vi "2D_tipconvolution.vi"() -> ()   [LabVIEW 2017]
uses:
  <vilib>/Analysis/2dsp.llb/2D Real FFT.vi
  <vilib>/Analysis/2dsp.llb/2D Inverse Real FFT.vi
  <vilib>/Analysis/NI_AALBase.lvlib
  <vilib>/Analysis/NI_AALPro.lvlib
panel:
  out "II tip sample convolution":dbl[][](graph)
  in  "index (row)":i32=18
  out "Sample crossections":dynamicdata(graph)
  out "tip sample convolution":dbl[][](graph)
  in  "tipangle":dbl=20.0 min=1.0 max=89.0 format="%.2f"
  in  "radius of curvature":dbl=10.0 min=-0.0 max=1000.0 format="%.2f"
  out "tipshape crossection horizontal":dbl[](graph)=[0.0, 0.0, 0.0, 0.0, 0.0, 0.0, 0.0, 0.0, 0.0, 0.0, 0.0, 0.0, 0.0, 0.0, 0.0, 0.0, 0.0, 0.0, 0.0, 0.0, 0.0, 0.0, 0.0, 0.0, 0.0, 0.0, 0.0, 0.0, 0.0, 0.0, 0.0, 0.0, 0.0, 0.0, 0.0, 0.0, 0.0, 0.0, 0.0, 0.0, 0.0, 0.0, 0.0, 0.0, 0.0, 0.0, 0.0, 0.0, 0.0, 0.0, 0.0, 0.0, 0.0, 0.0, 0.0, 0.0, 0.0, 0.0, 0.0, 0.0, 0.0, 0.0, 0.0, 0.0, 0.0, 0.0, 0.0, 0.0, 0.0, 0.0, 0.0, 0.0, 0.0, 0.0, 0.0, 0.0, 0.0, 0.0, 0.0, 0.0, 0.0, 0.0, 0.0, 0.0, 0.0, 0.0, 0.0, 0.0, 0.0, 0.0, 0.0, 0.0, 0.0, 0.0, 0.0, 0.0, 0.0, 0.0, 0.0, 0.0, 0.0, 0.0, 0.0, 0.0, 0.0, 0.0, 0.0, 0.0, 0.0, 0.0, 0.0, 0.0, 0.0, 0.0, 0.0, 0.0, 0.0, 0.0, 0.0, 0.0, 0.0, 0.0, 0.0, 0.0, 0.0, 0.0, 0.0, 0.0, 0.0, 0.0, 0.0, 0.0, 0.0, 0.0, 0.0, 0.0, 0.0, 0.0, 0.0, 0.0, 0.0, 0.0, 0.0, 0.0, 0.0, 0.0, 0.0, 0.0, 0.0, 0.0, 0.0, 0.0, 0.0, 0.0, 0.0, 0.0, 0.0, 0.0, 0.0, 0.0, 0.0, 0.0, 0.0, 0.0, 0.0, 0.0, 0.0, 0.0, 0.0, 0.0, 0.0, 0.0, 0.0, 0.0, 0.0, 0.0, 0.0, 0.0, 0.0, 0.0, 0.0, 0.0, 0.0, 0.0, 0.0, 0.0, 0.0, 0.0, 0.0, 0.0, 0.0, 0.0, 0.0, 0.0, 0.0, 0.0, 0.0, 0.0, 0.0, 0.0, 0.0, 0.0, 0.0, 0.0, 0.0, 0.0, 0.0, 0.0, 0.0, 0.0, 0.0, 0.0, 0.0, 0.0, 0.0, 0.0, 0.0, 0.0, 0.0, 0.0, 0.0, 0.0, 0.0, 0.0, 0.0, 0.0, 0.0, 0.0, 0.0, 0.0, 0.0, 0.0, 0.0, 0.0, 0.0, 0.0, 0.0, 0.0, 0.0, 1.7632698070846526, 4.358898943540674, 6.0, 7.14142842854285, 8.0, 8.660254037844387, 9.16515138991168, 9.539392014169456, 9.797958971132712, 9.9498743710662, 10.0, 9.9498743710662, 10.0, 9.9498743710662, 9.797958971132712, 9.539392014169456, 9.16515138991168, 8.660254037844387, 8.0, 7.14142842854285, 6.0, 4.358898943540674, 1.7632698070846526, 0.0, 0.0, 0.0, 0.0, 0.0, 0.0, 0.0, 0.0, 0.0, 0.0, 0.0, 0.0, 0.0, 0.0, 0.0, 0.0, 0.0, 0.0, 0.0, 0.0, 0.0, 0.0, 0.0, 0.0, 0.0, 0.0, 0.0, 0.0, 0.0, 0.0, 0.0, 0.0, 0.0, 0.0, 0.0, 0.0, 0.0, 0.0, 0.0, 0.0, 0.0, 0.0, 0.0, 0.0, 0.0, 0.0, 0.0, 0.0, 0.0, 0.0, 0.0, 0.0, 0.0, 0.0, 0.0, 0.0, 0.0, 0.0, 0.0, 0.0, 0.0, 0.0, 0.0, 0.0, 0.0, 0.0, 0.0, 0.0, 0.0, 0.0, 0.0, 0.0, 0.0, 0.0, 0.0, 0.0, 0.0, 0.0, 0.0, 0.0, 0.0, 0.0, 0.0, 0.0, 0.0, 0.0, 0.0, 0.0, 0.0, 0.0, 0.0, 0.0, 0.0, 0.0, 0.0, 0.0, 0.0, 0.0, 0.0, 0.0, 0.0, 0.0, 0.0, 0.0, 0.0, 0.0, 0.0, 0.0, 0.0, 0.0, 0.0, 0.0, 0.0, 0.0, 0.0, 0.0, 0.0, 0.0, 0.0, 0.0, 0.0, 0.0, 0.0, 0.0, 0.0, 0.0, 0.0, 0.0, 0.0, 0.0, 0.0, 0.0, 0.0, 0.0, 0.0, 0.0, 0.0, 0.0, 0.0, 0.0, 0.0, 0.0, 0.0, 0.0, 0.0, 0.0, 0.0, 0.0, 0.0, 0.0, 0.0, 0.0, 0.0, 0.0, 0.0, 0.0, 0.0, 0.0, 0.0, 0.0, 0.0, 0.0, 0.0, 0.0, 0.0, 0.0, 0.0, 0.0, 0.0, 0.0, 0.0, 0.0, 0.0, 0.0, 0.0, 0.0, 0.0, 0.0, 0.0, 0.0, 0.0, 0.0, 0.0, 0.0, 0.0, 0.0, 0.0, 0.0, 0.0, 0.0, 0.0, 0.0, 0.0, 0.0, 0.0, 0.0, 0.0, 0.0, 0.0, 0.0, 0.0, 0.0, 0.0, 0.0, 0.0, 0.0, 0.0, 0.0, 0.0, 0.0, 0.0, 0.0, 0.0, 0.0, 0.0, 0.0, 0.0, 0.0, 0.0, 0.0, 0.0, 0.0, 0.0, 0.0, 0.0, 0.0, 0.0, 0.0, 0.0, 0.0, 0.0, 0.0, 0.0, 0.0, 0.0, 0.0, 0.0, 0.0]
  out "block pattern like the NT-MDT TGQ01":dbl[][](graph)
  in  "cycles y":dbl=5.0 format="%0.2f"
  in  "pixels y":i32=500
  in  "cycles x":dbl=3.0 format="%0.2f"
  in  "pixels x":i32=500
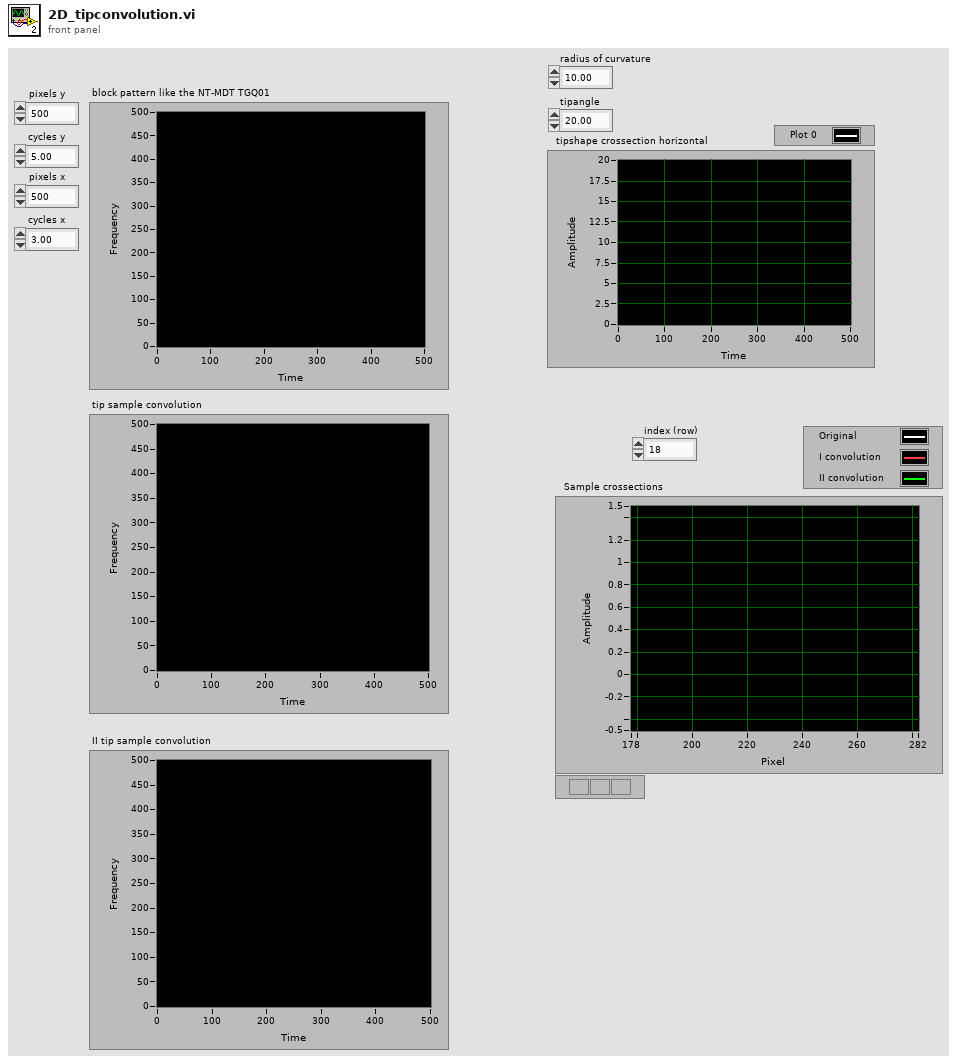
[diagram p1: front panel]
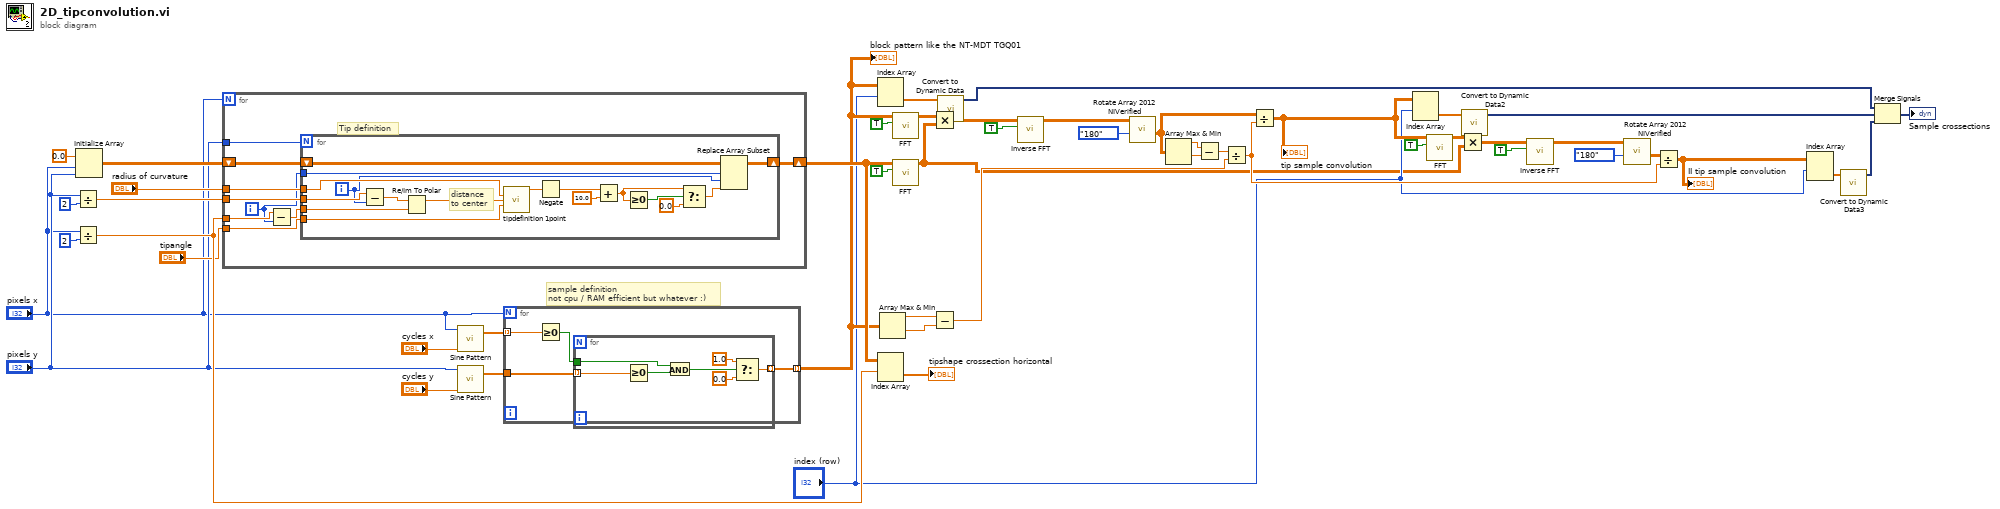
[diagram p0: block diagram]
diagram:
  # "sample definition\nnot cpu / RAM efficient but whatever :)"
  n1 = Divide(x="pixels y", y=2) -> (x/y=w44:dbl)
  n2 = Divide(x="pixels x", y=2) -> (x/y=w43:dbl)
  n3 = Initialize Array(0.0 ("element"), "pixels x", "pixels y") -> (w39:dbl[][])
  n4 = for {
    N: "pixels x" -> [_]
    tunnel: "pixels y" -> [w59]
    tunnel: w43 -> [w57]
    tunnel: w44 -> [w58]
    tunnel: "radius of curvature" -> [w56]
    tunnel: "tipangle" -> [w55]
    shift-right: [w53] -> w33
    shift-left: w39 -> [w54]
    i -> [w52]
    # "Tip definition"
    n5 = Subtract(x=w57, y=w52) -> (x-y=w51:dbl)
    n6 = for {
      N: w59 -> [_]
      tunnel: w58 -> [w76]
      tunnel: w56 -> [w75]
      tunnel: w55 -> [w74]
      shift-right: [w73] -> w53
      shift-left: w54 -> [w72]
      tunnel: w52 -> [w70]
      tunnel: w51 -> [w68]
      i -> [w71]
      # "distance\nto center"
      n7 = Subtract(x=w76, y=w71) -> (x-y=w69:dbl)
      n8 = Re/Im To Polar(2:w68, 3:w69) -> (1:w67:dbl)  [unwired: 1 out]
      n9 = call "tipdefinition 1point.vi"("radius of curvature"=w75, "x"=w67, "tipangle"=w74) -> ("result"=w66:dbl)  [unwired: 12 in]
      n10 = Negate(x=w66) -> (-x=w65:dbl)
      n11 = Add(x=w65, y=10.0) -> (x+y=w62:dbl)
      n12 = Greater Or Equal To 0?(x=w62) -> (x >= 0?=w63:bool)
      n13 = Select(t=w62, s=w63, f=0.0) -> (s? t:f=w60:dbl)
      n14 = Replace Array Subset(array=w72, new element=w60, index (row)=w70, index (col)=w71) -> (w73:dbl[][])
    }
  }
  n15 = call <vilib>:"Sine Pattern.vi"("cycles"="cycles x", "samples"="pixels x") -> ("Sinusoidal Pattern"=w47:dbl[])  [unwired: 2 in, 1 out]
  n16 = call <vilib>:"Sine Pattern.vi"("cycles"="cycles y", "samples"="pixels y") -> ("Sinusoidal Pattern"=w48:dbl[])  [unwired: 2 in, 1 out]
  n17 = for {
    N: "pixels x" -> [_]
    tunnel: w48 -> [w77]
    tunnel: w47 -> [w79] mode=indexing
    tunnel: [w80] -> w16 mode=indexing
    n18 = Greater Or Equal To 0?(x=w79) -> (x >= 0?=w78:bool)
    n19 = for {
      tunnel: w77 -> [w87] mode=indexing
      tunnel: [w84] -> w80 mode=indexing
      tunnel: w78 -> [w83]
      n20 = Greater Or Equal To 0?(x=w87) -> (x >= 0?=w82:bool)
      n21 = And(x=w83, y=w82) -> (x .and. y?=w81:bool)
      n22 = Select(t=1.0, s=w81, f=0.0) -> (s? t:f=w84:dbl)
    }
  }
  "block pattern like the NT-MDT TGQ01" <- w16
  n23 = Index Array(array=w16, index (row)="index (row)") -> (element=w15:dbl[])  [unwired: 1 in]
  n24 = Index Array(array=w33, index (row)=w43) -> (element=→"tipshape crossection horizontal":dbl[])  [unwired: 1 in]
  n25 = Array Max & Min(array=w16) -> (max value=w27:dbl, min value=w26:dbl)  [unwired: 2 out]
  n26 = call-poly <vilib>:"FFT.vi"("shift?"=TRUE, "X"=w16) -> ("FFT {X}"=w35:cdb[][])  [unwired: 8 in, 1 out]
  n27 = call-poly <vilib>:"FFT.vi"("shift?"=TRUE, "X"=w33) -> ("FFT {X}"=w1:cdb[][])  [unwired: 8 in, 1 out]
  n28 = Multiply(x=w35, y=w1) -> (x*y=w34:cdb[][])
  n29 = Subtract(x=w27, y=w26) -> (x-y=w22:dbl)
  n30 = call "Convert to Dynamic Data"("Array"=w15) -> ("Dynamic Data Type"=w14:dynamicdata)  [unwired: 3 in]
  n31 = call-poly <vilib>:"Inverse FFT.vi"("shift?"=TRUE, "FFT {X}"=w34) -> ("X"=w29:dbl[][])  [unwired: 8 in, 1 out]
  n32 = call "Rotate Array 2012 NIVerified.vi"("Rotation"=enum8{"90", "180", "270"}."180", "Array"=w29) -> ("Rotated 2D Array"=w3:dbl[][])  [unwired: 9 in]
  n33 = Array Max & Min(array=w3) -> (max value=w25:dbl, min value=w24:dbl)  [unwired: 2 out]
  n34 = Subtract(x=w25, y=w24) -> (x-y=w23:dbl)
  n35 = Divide(x=w23, y=w22) -> (x/y=w18:dbl)
  n36 = Divide(x=w3, y=w18) -> (x/y=w12:dbl[][])
  "tip sample convolution" <- w12
  n37 = Index Array(array=w12, index (row)="index (row)") -> (element=w11:dbl[])  [unwired: 1 in]
  n38 = call-poly <vilib>:"FFT.vi"("shift?"=TRUE, "X"=w12) -> ("FFT {X}"=w20:cdb[][])  [unwired: 8 in, 1 out]
  n39 = Multiply(x=w20, y=w1) -> (x*y=w6:cdb[][])
  n40 = call "Convert to Dynamic Data2"("Array"=w11) -> ("Dynamic Data Type"=w10:dynamicdata)  [unwired: 3 in]
  n41 = call-poly <vilib>:"Inverse FFT.vi"("shift?"=TRUE, "FFT {X}"=w6) -> ("X"=w5:dbl[][])  [unwired: 8 in, 1 out]
  n42 = call "Rotate Array 2012 NIVerified.vi"("Rotation"=enum8{"90", "180", "270"}."180", "Array"=w5) -> ("Rotated 2D Array"=w2:dbl[][])  [unwired: 9 in]
  n43 = Divide(x=w2, y=w18) -> (x/y=w4:dbl[][])
  "II tip sample convolution" <- w4
  n44 = Index Array(array=w4, index (row)="index (row)") -> (element=w8:dbl[])  [unwired: 1 in]
  n45 = call "Convert to Dynamic Data3"("Array"=w8) -> ("Dynamic Data Type"=w7:dynamicdata)  [unwired: 3 in]
  n46 = Merge Signals(w14, w10, w7) -> (→"Sample crossections":dynamicdata)
